vi "AddFailure_WithGrandparent_GrandparentFailureIconSet.vi"() -> (0 "error out":errorcluster)   [LabVIEW 2017, in "ResultTreeListener.Tests.lvlib"]
uses:
  ResultTreeListener.Tests.lvlib
  ResultTree/Icon.ctl
  275d98eb-69a7-4435-8809-2af3ffd1cf1d.vi
  Support/FakeTestCase/FakeTestCase.lvclass
  C:/Users/de200256/Code/logmanoriginal/lvunit/Test/Test.lvclass
  Support/FakeTestSuite/FakeTestSuite.lvclass
  C:/Users/de200256/Code/logmanoriginal/lvunit/TestSuite/TestSuite.lvclass
  Constraint/IsEqual/Create.vi
  ResultTreeListener/ResultTreeListener.lvclass
  Constraint/IsEqual/IsEqual.lvclass
  ResultTree/ResultTree.lvclass
panel:
  in  "Tree":string(tree)
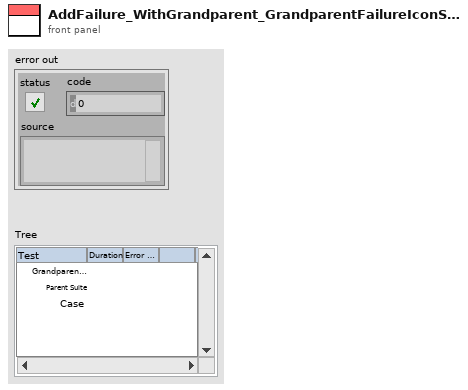
[diagram p1: front panel]
types:
  T1 = typedef "ResultTree.lvclass/Icon.ctl" = enum16{"None", "Passed", "Failed", "Error"}
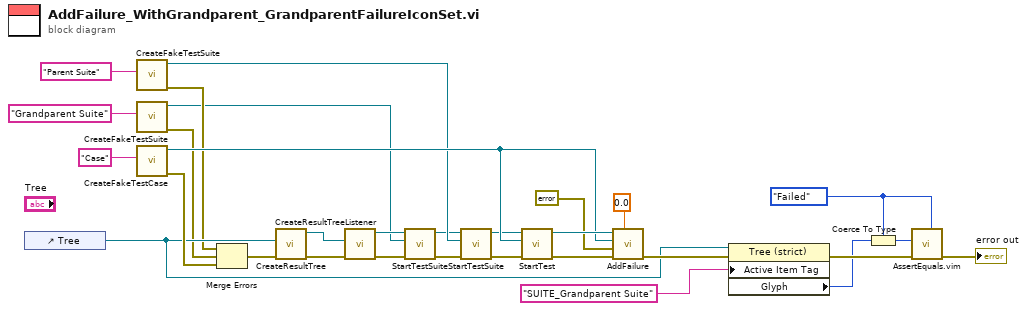
[diagram p0: block diagram]
diagram:
  w14 = Icon."Failed" ("Active Cell:String")
  n1 = control-ref of="Tree"() -> (w19:refnum<vi>)
  n2 = call "CreateFakeTestSuite.vi"("Name"="Parent Suite") -> ("error out"=w6:errorcluster, "FakeTestSuite out"=w9:refnum<class "FakeTestSuite.lvclass">)  [unwired: 9 in]
  n3 = call "CreateFakeTestSuite.vi"("Name"="Grandparent Suite") -> ("error out"=w7:errorcluster, "FakeTestSuite out"=w1:refnum<class "FakeTestSuite.lvclass">)  [unwired: 9 in]
  n4 = call "CreateFakeTestCase.vi"("Name"="Case") -> ("error out"=w24:errorcluster, "FakeTestCase out"=w22:refnum<class "FakeTestCase.lvclass">)  [unwired: 9 in]
  n5 = Merge Errors(w6, w7, w24) -> (w12:errorcluster)
  n6 = call "CreateResultTree.vi"("error in (no error)"=w12, "Tree Refnum"=w19) -> ("error out"=w30:errorcluster, "ResultTree out"=w29:refnum<class "ResultTree.lvclass">)  [unwired: 8 in]
  n7 = call "CreateResultTreeListener.vi"("error in (no error)"=w30, "ResultTree"=w29) -> ("error out"=w5:errorcluster, "ResultTreeListener out"=w4:refnum<class "ResultTreeListener.lvclass">)  [unwired: 8 in]
  n8 = call-dynamic "StartTestSuite.vi"("error in (no error)"=w5, "TestSuite"=w1, "ResultTreeListener in"=w4) -> ("error out"=w2:errorcluster, "ResultTreeListener out"=w3:refnum<class "ResultTreeListener.lvclass">)  [unwired: 7 in]
  n9 = call-dynamic "StartTestSuite.vi"("error in (no error)"=w2, "TestSuite"=w9, "ResultTreeListener in"=w3) -> ("error out"=w11:errorcluster, "ResultTreeListener out"=w10:refnum<class "ResultTreeListener.lvclass">)  [unwired: 7 in]
  n10 = call-dynamic "StartTest.vi"("error in (no error)"=w11, "Test"=w22, "ResultTreeListener in"=w10) -> ("error out"=w26:errorcluster, "ResultTreeListener out"=w25:refnum<class "ResultTreeListener.lvclass">)  [unwired: 7 in]
  n11 = call-dynamic "AddFailure.vi"("Time"=0.0, "error in (no error)"=w26, "Failure"=errorcluster {"status"=FALSE, "code"=0, "source"=""}, "Test"=w22, "ResultTreeListener in"=w25) -> ("error out"=w23:errorcluster)  [unwired: 5 in, 1 out]
  n12 = property class="Tree (strict)"(reference=w19, error in=w23, "Active Item Tag"="SUITE_Grandparent Suite" ("Active Item:Tag")) -> (error out=w20:errorcluster, "Glyph"=w17:i32)  [unwired: 1 out]
  n13 = Coerce To Type(0:w17, 1:w14) -> (2:w15:T1)
  n14 = call "AssertEquals.vim"("Expected"=w14, "error in (no error)"=w20, "Actual"=w15) -> ("error out"=→"error out":errorcluster)  [unwired: 8 in]
